vi "delta test.vi"() -> ()   [LabVIEW 2020]
uses:
  DeltaTcp/DeltaTcp.lvclass
panel:
  out "data":i32[](array[numeric])
  out "Data":variant
  out "Data 2":variant
  in  "ipAddress":string="192.168.1.88"
  in  "station":u8=1
  in  "port":i32=502
  in  "series":i32(ring)=2 items=["DVP", "AS"]
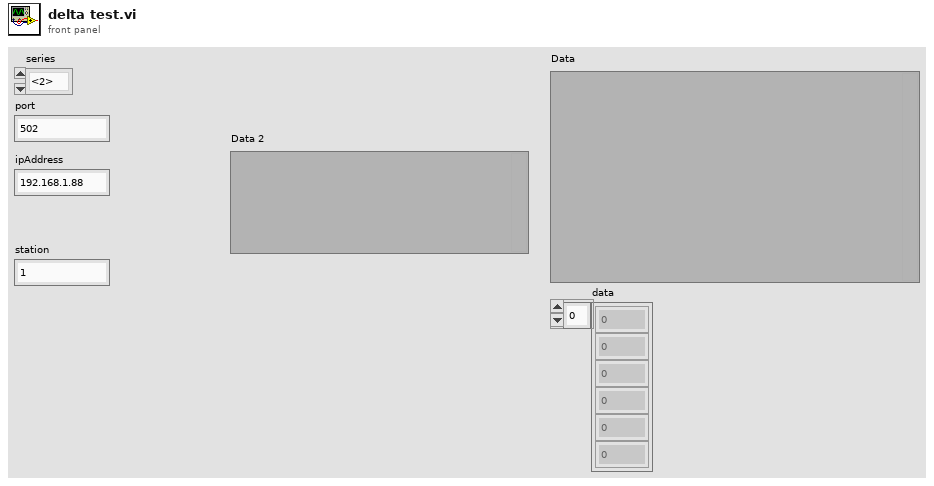
[diagram p1: front panel]
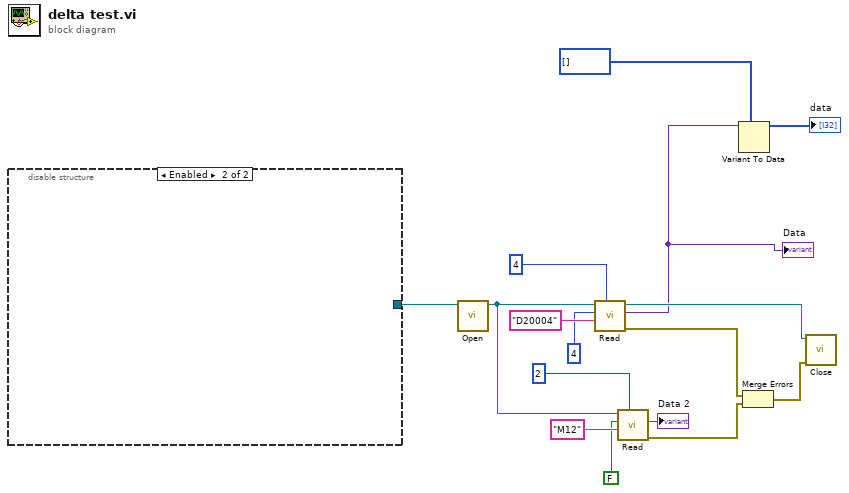
[diagram p0: block diagram]
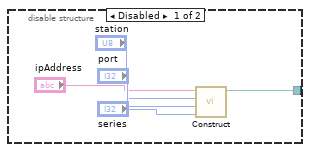
[diagram p2: hidden frame]
diagram:
  n1 = disable-structure shown="Enabled" {
    disable-tunnel: [w17 _] -> w16
    frame Disabled {
      n2 = call "Construct.vi"("series"="series", "port"="port", "station"="station", "ipAddress"="ipAddress") -> ("MelsecMcNet out"=w17:refnum<class "DeltaTcp.lvclass">)  [unwired: 7 in]
    }
    frame Enabled {
    }
  }
  n3 = call-dynamic "Open.vi"("MelsecTCP in"=w16) -> ("MelsecTCP out"=w11:refnum<class "DeltaTcp.lvclass">)  [unwired: 9 in, 1 out]
  n4 = call-dynamic "Read.vi"("length"=u16 4, "Start address"="D20004", "Read Type"=4 ("length"), "MelsecTCP in"=w11) -> ("error out"=w9:errorcluster, "Data"=w3:variant, "MelsecTCP out"=w10:refnum<class "DeltaTcp.lvclass">)  [unwired: 5 in]
  "Data" <- w3
  n5 = call-dynamic "Read.vi"("length"=u16 2, "Start address"="M12", "Read Type"=FALSE, "MelsecTCP in"=w11) -> ("error out"=w8:errorcluster, "Data"=→"Data 2":variant)  [unwired: 5 in, 1 out]
  n6 = Variant To Data(type=i32[] [] ("length"), Variant=w3) -> (data=→"data":i32[])  [unwired: 1 in, 1 out]
  n7 = Merge Errors(w9, w8) -> (w7:errorcluster)
  n8 = call-dynamic "Close.vi"("error in (no error)"=w7, "MelsecTCP in"=w10) -> ()  [unwired: 8 in, 2 out]
